vi "test_LoadCommandlineArgs_AddPackedLibWithPathCheckDefaults.vi"() -> (3 "Pass?":bool)   [LabVIEW 2019, in "Tests.SolutionBuilder.lvlib"]
uses:
  Tests.SolutionBuilder.lvlib
  SolutionBuilder/Community/Options.ctl
  SolutionBuilder/ProjectItem/ProjectItem.lvclass/ProjectItem.ctl
  SolutionBuilder/SolutionBuilder.lvclass
  SolutionBuilder/ProjectItem/ProjectItem.lvclass
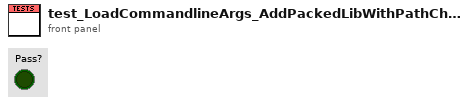
[diagram p1: front panel]
types:
  T1 = typedef "SolutionBuilder.lvlib/SolutionBuilder.lvclass/Options.ctl" = cluster{"Path":path, "Preview?":bool, "Quiet?":bool, "Log file":path, "Success file":path, "Rebuild?":bool, "Keep split projects?":bool}
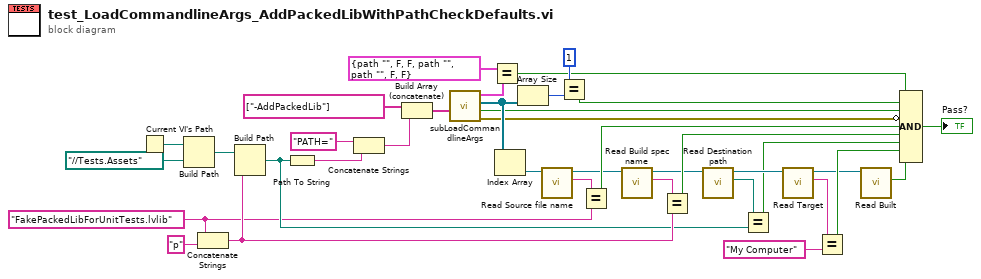
[diagram p0: block diagram]
diagram:
  w22 = "FakePackedLibForUnitTests.lvlib"
  n1 = Current VI's Path() -> (path=w11:path)
  n2 = Build Path(base path=w11, name or relative path=path "../../Tests.Assets" ("Path")) -> (appended path=w14:path)
  n3 = Concatenate Strings(w22, "p" ("string")) -> (w29:string)
  n4 = Build Path(base path=w14, name or relative path=w29) -> (appended path=w23:path)
  n5 = Path To String(path=w23) -> (string=w31:string)
  n6 = Concatenate Strings("PATH=" ("string"), w31) -> (w32:string)
  n7 = Build Array (concatenate)(string[] ["-AddPackedLib"] ("App.Args"), w32) -> (w12:string[])
  n8 = call "subLoadCommandlineArgs.vi"("App.Args"=w12) -> ("error out"=w5:errorcluster, "From command line?"=w1:bool, "Pre-built libraries"=w13:refnum<class "ProjectItem.lvclass">[], "Options"=w3:T1)  [unwired: 6 in, 1 out]
  n9 = Equal?(x=T1 {"Path"=path "", "Preview?"=FALSE, "Quiet?"=FALSE, "Log file"=path "", "Success file"=path "", "Rebuild?"=FALSE, "Keep split projects?"=FALSE} ("Options"), y=w3) -> (x = y?=w2:bool)
  n10 = Index Array(array=w13) -> (element=w15:refnum<class "ProjectItem.lvclass">)  [unwired: 1 in]
  n11 = Array Size(array=w13) -> (size(s)=w6:i32)
  n12 = call "Read Source file name.vi"("ProjectItem in"=w15) -> ("Source file name"=w20:string, "ProjectItem out"=w17:refnum<class "ProjectItem.lvclass">)  [unwired: 9 in]
  n13 = Equal?(x=1, y=w6) -> (x = y?=w8:bool)
  n14 = Equal?(x=w20, y=w22) -> (x = y?=w25:bool)
  n15 = call "Read Build spec name.vi"("ProjectItem in"=w17) -> ("Build spec name"=w21:string, "ProjectItem out"=w18:refnum<class "ProjectItem.lvclass">)  [unwired: 9 in]
  n16 = Equal?(x=w21, y=w29) -> (x = y?=w26:bool)
  n17 = call "Read Destination path.vi"("ProjectItem in"=w18) -> ("Destination path"=w24:path, "ProjectItem out"=w33:refnum<class "ProjectItem.lvclass">)  [unwired: 9 in]
  n18 = Equal?(x=w24, y=w23) -> (x = y?=w27:bool)
  n19 = call "Read Target.vi"("ProjectItem in"=w33) -> ("Target"=w35:string, "ProjectItem out"=w34:refnum<class "ProjectItem.lvclass">)  [unwired: 9 in]
  n20 = Equal?(x=w35, y="My Computer") -> (x = y?=w37:bool)
  n21 = call "Read Built.vi"("ProjectItem in"=w34) -> ("Built"=w19:bool)  [unwired: 9 in, 1 out]
  n22 = Compound Arithmetic op=AND(w2, w8, w1, invert w5, w25, w26, w27, w37, w19) -> (→"Pass?":bool)
